vi "S2C_FORNAX_Proc_ViperRequest.vi"(7 "Local?":bool, 8 "Error In":errorcluster, 9 "CmdString":string, 10 "Command":string, 11 "Timeout":dbl) -> (0 "Error Out":errorcluster, 3 "Response":string)   [LabVIEW 2015]
uses:
  S2C_FORNAX_Proc_Globals.vi
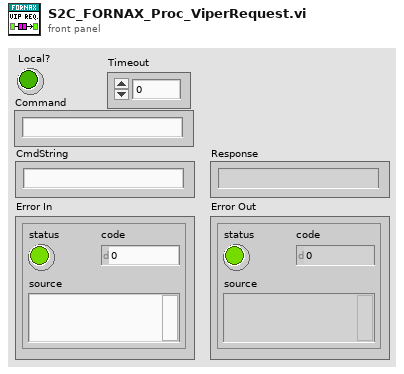
[diagram p1: front panel]
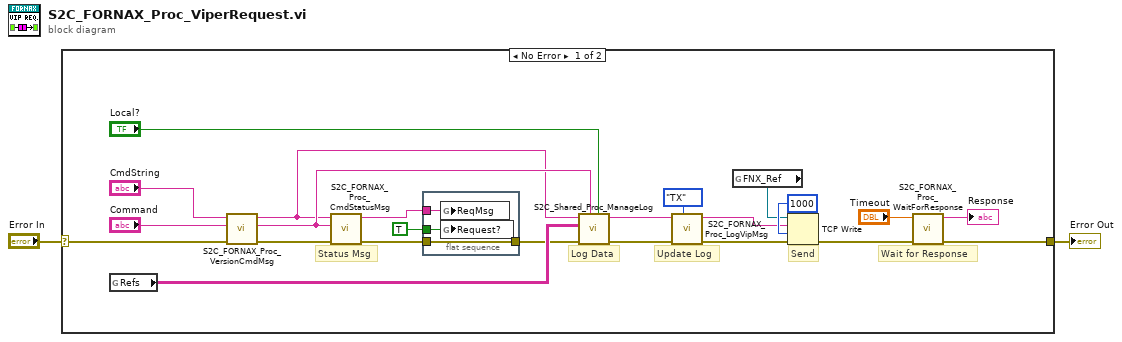
[diagram p0: block diagram]
diagram:
  n1 = case shown="No Error" "Error In" {
    selector: "Error In" -> [w8 w29]
    tunnel: [w17 w29] -> w1
    frame No Error {
      # "Log Data"
      # "Update Log"
      # "Wait for Response"
      # "Status Msg"
      # "Send"
      n2 = global read "S2C_FORNAX_Proc_Globals.vi" "Refs"() -> (w11:string[][])
      n3 = call "S2C_FORNAX_Proc_VersionCmdMsg.vi"("Error In"=w8, "Cmd In"="Command", "JSON In"="CmdString") -> ("Error Out"=w7:errorcluster, "Cmd Out"=w4:string, "JSON Out"=w3:string)  [unwired: 6 in]
      n4 = call "S2C_FORNAX_Proc_CmdStatusMsg.vi"("Error In"=w7, "CmdMsg"=w4, "CmdString"=w3) -> ("Error Out"=w24:errorcluster, "StatusMsg"=w23:string)  [unwired: 7 in]
      n5 = flat-sequence {
        tunnel: w24 -> [w28]
        tunnel: [w28] -> w9
        tunnel: w23 -> [w27]
        tunnel: TRUE ("Request?") -> [w26]
        frame #0 {
          n6 = global write "S2C_FORNAX_Proc_Globals.vi" "ReqMsg"(w27) -> ()
          n7 = global write "S2C_FORNAX_Proc_Globals.vi" "Request?"(w26) -> ()
        }
      }
      n8 = call "S2C_Shared_Proc_ManageLog.vi"("Local?"="Local?", "Command"=w4, "Error In"=w9, "Refs"=w11, "Data In"=w3) -> ("Error Out"=w10:errorcluster, "Data Out"=w13:string)  [unwired: 5 in]
      n9 = call "S2C_FORNAX_Proc_LogVipMsg.vi"("Direction"=enum16{"TX", "RX"}."TX", "Error In"=w10, "Msg In"=w13) -> ("Error Out"=w14:errorcluster, "Msg Out"=w15:string)  [unwired: 7 in]
      n10 = global read "S2C_FORNAX_Proc_Globals.vi" "FNX_Ref"() -> (w19:refnum<k5>)
      n11 = TCP Write(connection ID=w19, data in=w15, error in (no error)=w14, 9:1000 ("timeout ms (25000)")) -> (error out=w21:errorcluster)  [unwired: 2 out]
      n12 = call "S2C_FORNAX_Proc_WaitForResponse.vi"("Error In"=w21, "Timeout"="Timeout") -> ("Error Out"=w17:errorcluster, "Response"=→"Response":string)  [unwired: 8 in]
    }
    frame Error {
    }
  }
  "Error Out" <- w1
